vi "Modbus Kommunikation.vi"(4 "VISA resource in":refnum<visa-resource-name>, 6 "Data In / #Reads [U16]":u16[](array[numeric]), 7 "Modbus Port (Port,  Baudrate)":T1={"COM Port"="COM3", "Baud Rate"=9600}, 8 "error in (no error)":errorcluster, 9 "Register Start Address":u16 format="%x", 10 "Slave Address":u8, 11 "Command":T2) -> (0 "error out":errorcluster, 1 "Data Out [U16]":u16[](array[numeric]), 3 "VISA resource out":refnum<visa-resource-name>)   [LabVIEW 2024, in "Voegtlin_NI_SMART_Modbus_Drivers.lvlib"]
doc: "Fuehrt Modbus-Kommunikation gemaess Command aus."
uses:
  Voegtlin_NI_SMART_Modbus_Drivers.lvlib
  Enums/Modbus Comm.ctl
  Port.ctl
  Sotronik_Modbus_Serial_Master.llb/Modbus_Command.ctl
  Sotronik_Modbus_Serial_Master.llb/Modbus_Connection_Data.ctl
panel:
  # "Input Data"
  # "Internal Data"
  # "Output Data"
  # "(Inputmaske in HEX)"
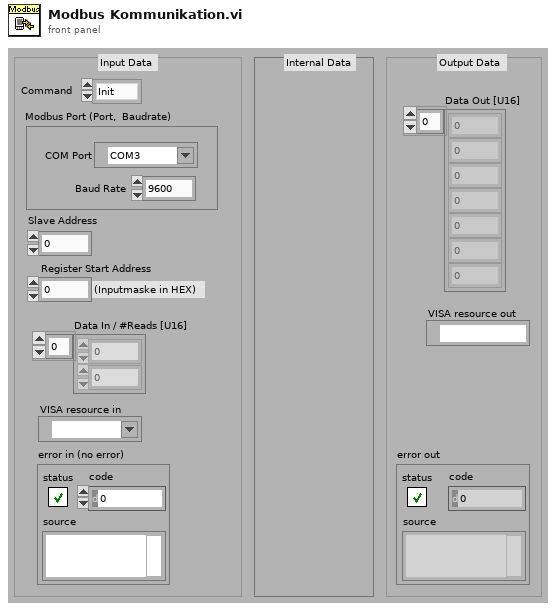
[diagram p1: front panel]
types:
  T1 = typedef "Voegtlin_NI_SMART_Modbus_Drivers.lvlib/Port.ctl" = cluster{"COM Port":refnum<visa-resource-name>, "Baud Rate":u32}
  T2 = typedef "Voegtlin_NI_SMART_Modbus_Drivers.lvlib/Modbus Comm.ctl" = enum16{"Init", "Read", "Write", "Exit"}
  T3 = cluster{"Timeout":u32, "Flow Control":u16, "Parity":u16, "Mode":enum16{"RTU", "ASCII"}}
  T4 = typedef "Voegtlin_NI_SMART_Modbus_Drivers.lvlib/Modbus_Connection_Data.ctl" = cluster{"VISA resource name out":refnum<visa-resource-name>, "Mode":enum16{"RTU", "ASCII"}, "Timeout":u32}
  T5 = typedef "Voegtlin_NI_SMART_Modbus_Drivers.lvlib/Modbus_Command.ctl" = cluster{"Starting Address":u16, "Quantity":u16, "Slave Address":u8, "Function Code":u8}
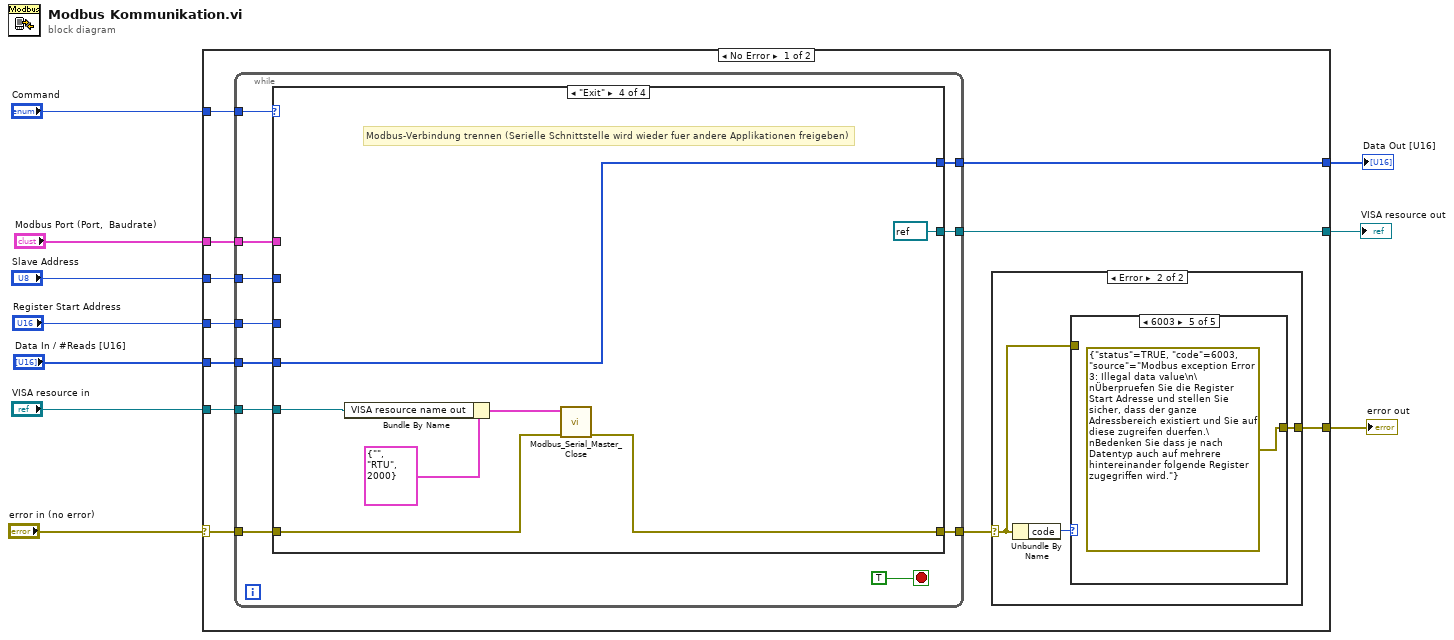
[diagram p0: block diagram]
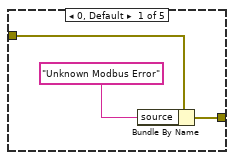
[diagram p3: hidden frame]
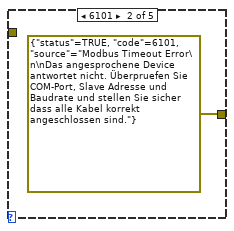
[diagram p4: hidden frame]
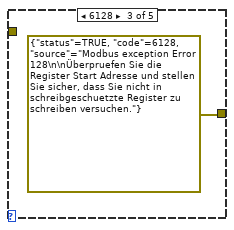
[diagram p5: hidden frame]
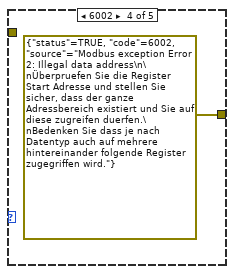
[diagram p6: hidden frame]
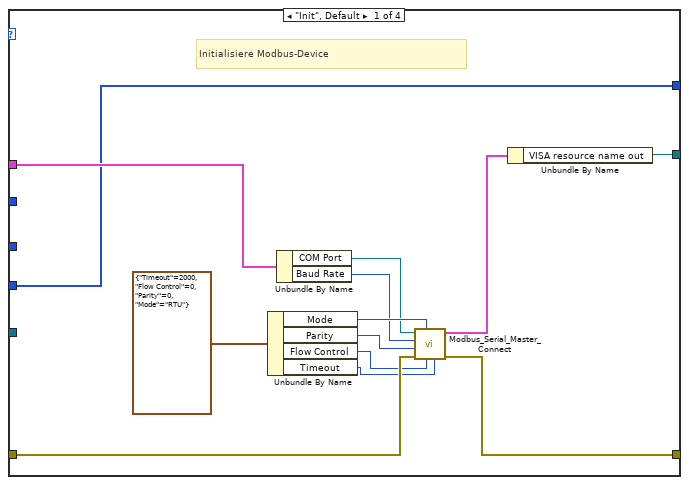
[diagram p7: hidden frame]
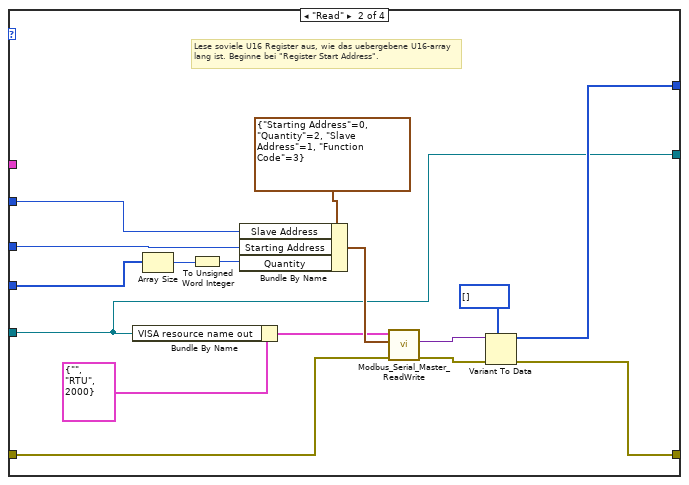
[diagram p8: hidden frame]
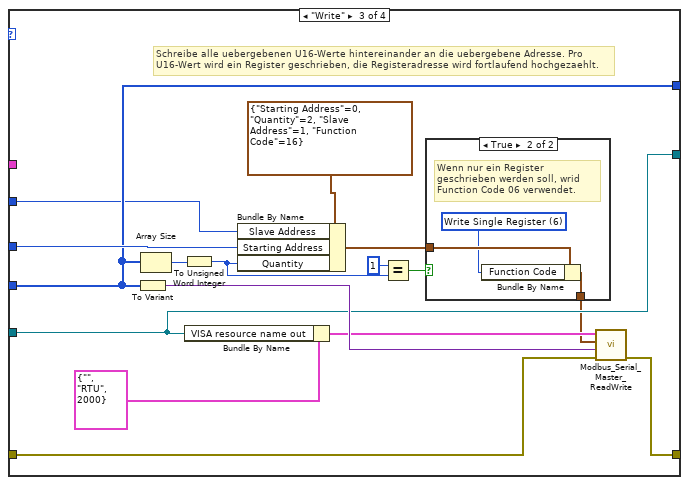
[diagram p9: hidden frame]
diagram:
  n1 = case shown="No Error" "error in (no error)" {
    selector: "error in (no error)" -> [w20 w102]
    tunnel: [w14 w102] -> w9
    tunnel: "Command" -> [w21 _]
    tunnel: "Modbus Port (Port,  Baudrate)" -> [w19 _]
    tunnel: "Data In / #Reads [U16]" -> [w18 w101]
    tunnel: "Register Start Address" -> [w17 _]
    tunnel: [w16 w101] -> w5
    tunnel: "Slave Address" -> [w13 _]
    tunnel: [w12 w100] -> w2
    tunnel: "VISA resource in" -> [w11 w100]
    frame No Error {
      n2 = while {
        tunnel: w21 -> [w43]
        tunnel: w20 -> [w42]
        tunnel: [w40] -> w15
        tunnel: w19 -> [w39]
        tunnel: w18 -> [w38]
        tunnel: w17 -> [w37]
        tunnel: [w36] -> w16
        tunnel: w13 -> [w35]
        tunnel: [w34] -> w12
        tunnel: w11 -> [w33]
        stop <- TRUE stop-if-true
        n3 = case shown="\"Exit\"" w43 {
          tunnel: w42 -> [w54 w72 w87 w99]
          tunnel: w33 -> [_ w57 w78 w95]
          tunnel: [w56 w69 w82 w98] -> w40
          tunnel: w39 -> [w52 _ _ _]
          tunnel: w38 -> [w51 w68 w83 w97]
          tunnel: w37 -> [_ w63 w84 _]
          tunnel: [w51 w62 w83 w97] -> w36
          tunnel: w35 -> [_ w60 w81 _]
          tunnel: [w44 w57 w78 refnum<visa-resource-name> refnum ("VISA resource in")] -> w34
          frame "Init", Default {
            # "Initialisiere Modbus-Device"
            n4 = Unbundle By Name(T3 {"Timeout"=2000, "Flow Control"=0, "Parity"=0, "Mode"=enum."RTU"}) -> ("Mode"=w55:enum16{"RTU", "ASCII"}, "Parity"=w48:u16, "Flow Control"=w47:u16, "Timeout"=w46:u32)
            n5 = Unbundle By Name(w52) -> ("COM Port"=w53:refnum<visa-resource-name>, "Baud Rate"=w49:u32)
            n6 = call "Modbus_Serial_Master_Connect.vi"("Timeout"=w46, "Flow Control"=w47, "Mode"=w55, "error in (no error)"=w54, "Parity"=w48, "Baud Rate"=w49, "VISA resource name"=w53) -> ("error out"=w56:errorcluster, "Modbus Connection"=w45:T4)  [unwired: 3 in]
            n7 = Unbundle By Name(w45) -> ("VISA resource name out"=w44:refnum<visa-resource-name>)
          }
          frame "Read" {
            # "Lese soviele U16 Register aus, wie das uebergebene U16-array lang ist. Beginne bei \"Register Start Address\"."
            n8 = Bundle By Name(cluster=T4 {"VISA resource name out"="", "Mode"=enum."RTU", "Timeout"=2000} ("Modbus Connection"), "VISA resource name out"=w57) -> (w58:T4)
            n9 = Array Size(array=w68) -> (size(s)=w64:i32)
            n10 = To Unsigned Word Integer(number=w64) -> (unsigned 16bit integer=w61:u16)
            n11 = Bundle By Name(cluster=T5 {"Starting Address"=0, "Quantity"=2, "Slave Address"=1, "Function Code"=3} ("Modbus Command"), "Slave Address"=w60, "Starting Address"=w63, "Quantity"=w61) -> (w65:T5)
            n12 = call "Modbus_Serial_Master_ReadWrite.vi"("error IN"=w72, "Modbus Command"=w65, "Modbus Connection IN"=w58) -> ("error OUT"=w70:errorcluster, "Data Out"=w71:variant)  [unwired: 6 in, 1 out]
            n13 = Variant To Data(error in=w70, type=u16[] [], Variant=w71) -> (data=w62:u16[], error out=w69:errorcluster)
          }
          frame "Write" {
            # "Schreibe alle uebergebenen U16-Werte hintereinander an die uebergebene Adresse. Pro U16-Wert wird ein Register geschrieben, die Registeradresse wird fortlaufend hochgezaehlt."
            n14 = To Variant(anything=w83) -> (Variant=w88:variant)
            n15 = Array Size(array=w83) -> (size(s)=w85:i32)
            n16 = To Unsigned Word Integer(number=w85) -> (unsigned 16bit integer=w76:u16)
            n17 = Bundle By Name(cluster=T4 {"VISA resource name out"="", "Mode"=enum."RTU", "Timeout"=2000} ("Modbus Connection"), "VISA resource name out"=w78) -> (w79:T4)
            n18 = Bundle By Name(cluster=T5 {"Starting Address"=0, "Quantity"=2, "Slave Address"=1, "Function Code"=16} ("Modbus Command"), "Slave Address"=w81, "Starting Address"=w84, "Quantity"=w76) -> (w74:T5)
            n19 = Equal?(x=u16 1 ("y"), y=w76) -> (x = y?=w77:bool)
            n20 = case shown="True" w77 {
              tunnel: w74 -> [w89 w92]
              tunnel: [w89 w91] -> w73
              frame False {
              }
              frame True {
                w90 = u8 6 items=["Read Coils"=1, "Read Discrete Inputs"=2, "Read Holding Registers"=3, "Read Input Registers"=4, "Write Single Coil"=5, "Write Single Register"=6, "Read Exception Status"=7, "Write Multiple Coils"=15, "Write Multiple Registers"=16] ("Function Code")
                # "Wenn nur ein Register geschrieben werden soll, wrid Function Code 06 verwendet."
                n21 = Bundle By Name(cluster=w92, "Function Code"=w90) -> (w91:T5)
              }
            }
            n22 = call "Modbus_Serial_Master_ReadWrite.vi"("error IN"=w87, "Data IN"=w88, "Modbus Command"=w73, "Modbus Connection IN"=w79) -> ("error OUT"=w82:errorcluster)  [unwired: 5 in, 2 out]
          }
          frame "Exit" {
            # "Modbus-Verbindung trennen (Serielle Schnittstelle wird wieder fuer andere Applikationen freigeben)"
            n23 = Bundle By Name(cluster=T4 {"VISA resource name out"="", "Mode"=enum."RTU", "Timeout"=2000} ("Modbus Connection"), "VISA resource name out"=w95) -> (w93:T4)
            n24 = call "Modbus_Serial_Master_Close.vi"("error in (no error)"=w99, "Modbus Connection"=w93) -> ("error out"=w98:errorcluster)  [unwired: 9 in]
          }
        }
      }
      n25 = case shown="Error" w15 {
        selector: w15 -> [w22 w23]
        tunnel: [w22 w24] -> w14
        frame No Error {
        }
        frame Error {
          n26 = Unbundle By Name(w23) -> ("code"=w25:i32)
          n27 = case shown="6003" w25 {
            tunnel: [w27 errorcluster {"status"=TRUE, "code"=6101, "source"="Modbus Timeout Error\n\nDas angesprochene Device antwortet nicht. Überpruefen Sie COM-Port, Slave Adresse und Baudrate und stellen Sie sicher dass alle Kabel korrekt angeschlossen sind."} ("error IO") errorcluster {"status"=TRUE, "code"=6128, "source"="Modbus exception Error 128\n\nÜberpruefen Sie die Register Start Adresse und stellen Sie sicher, dass Sie nicht in schreibgeschuetzte Register zu schreiben versuchen."} ("error IO") errorcluster {"status"=TRUE, "code"=6002, "source"="Modbus exception Error 2: Illegal data address\n\nÜberpruefen Sie die Register Start Adresse und stellen Sie sicher, dass der ganze Adressbereich existiert und Sie auf diese zugreifen duerfen.\nBedenken Sie dass je nach Datentyp auch auf mehrere hintereinander folgende Register zugegriffen wird."} ("error IO") errorcluster {"status"=TRUE, "code"=6003, "source"="Modbus exception Error 3: Illegal data value\n\nÜberpruefen Sie die Register Start Adresse und stellen Sie sicher, dass der ganze Adressbereich existiert und Sie auf diese zugreifen duerfen.\nBedenken Sie dass je nach Datentyp auch auf mehrere hintereinander folgende Register zugegriffen wird."} ("error IO")] -> w24
            tunnel: w23 -> [w28 _ _ _ _]
            frame 0, Default {
              n28 = Bundle By Name(cluster=w28, "source"="Unknown Modbus Error") -> (w27:errorcluster)
            }
            frame 6101 {
            }
            frame 6128 {
            }
            frame 6002 {
            }
            frame 6003 {
            }
          }
        }
      }
    }
    frame Error {
    }
  }
  "error out" <- w9
  "Data Out [U16]" <- w5
  "VISA resource out" <- w2
